vi "Get FC1.vi"(11 "SingleCylinderActuator in":refnum<class "Dual Cylinder Actuator.lvclass">) -> (2 "FC1":refnum<class "Actuator Cylinder.lvclass">, 3 "SingleCylinderActuator out":refnum<class "Dual Cylinder Actuator.lvclass">)   [LabVIEW 2015, in "Dual Cylinder Actuator.lvclass"]
uses:
  Dual Cylinder Actuator.lvclass
  Actuator Cylinder/Actuator Cylinder/Actuator Cylinder.lvclass
  Dual Cylinder Actuator.lvclass/Dual Cylinder Actuator.ctl
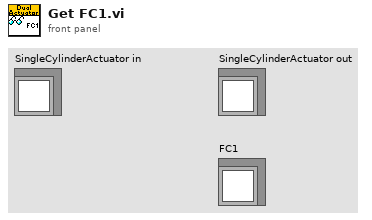
[diagram p1: front panel]
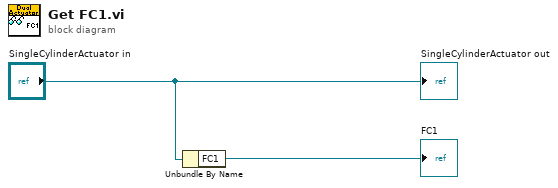
[diagram p0: block diagram]
diagram:
  n1 = Unbundle By Name("SingleCylinderActuator in") -> ("FC1"=→"FC1":refnum<class "Actuator Cylinder.lvclass">)
  "SingleCylinderActuator out" <- "SingleCylinderActuator in"
